vi "Receive mDNS Response.vi"(7 "timeout, ms (5000)":i32=5000, 8 "error in (no error)":errorcluster, 10 "query id":u16, 11 "connection ID":refnum<k16>) -> (0 "error out":errorcluster, 2 "response":T1 {"header"."response code" items=["NoError"=0, "FormErr"=1, "ServFail"=2, "NXDomain"=3, "NotImp"=4, "Refused"=5, "YXDomain"=6, "YXRRSet"=7, "NXRRSet"=8, "NotAuth"=9, "NotZone"=10, "DSOTYPENI"=11, "BADVERS/BADSIG"=16, "BADKEY"=17, "BADTIME"=18, "BADMODE"=19, "BADNAME"=20, "BADALG"=21, "BADTRUNC"=22, "BADCOOKIE"=23]; "header"."opcode" items=["Query"=0, "IQuery"=1, "Status"=2, "Notify"=4, "Update"=5, "DSO"=6]; "additional records"."class" items=["IN"=1, "CH"=3, "HS"=4]; "additional records"."type" items=["A"=1, "NS"=2, "MD"=3, "MF"=4, "CNAME"=5, "SOA"=6, "MB"=7, "MG"=8, "MR"=9, "NULL"=10, "WKS"=11, "PTR"=12, "HINFO"=13, "MINFO"=14, "MX"=15, "TXT"=16, "RP"=17, "AFSDB"=18, "X25"=19, "ISDN"=20, "RT"=21, "NSAP"=22, "NSAP-PTR"=23, "SIG"=24, "KEY"=25, "PX"=26, "GPOS"=27, "AAAA"=28, "LOC"=29, "NXT"=30, "EID"=31, "NIMLOC"=32, "SRV"=33, "ATMA"=34, "NAPTR"=35, "KX"=36, "CERT"=37, "A6"=38, "DNAME"=39, "SINK"=40, "OPT"=41, "APL"=42, "DS"=43, "SSHFP"=44, "IPSECKEY"=45, "RRSIG"=46, "NSEC"=47, "DNSKEY"=48, "DHCID"=49, "NSEC3"=50, "NSEC3PARAM"=51, "TLSA"=52, "SMIMEA"=53, "HIP"=55, "NINFO"=56, "RKEY"=57, "TALINK"=58, "CDS"=59, "CDNSKEY"=60, "OPENPGPKEY"=61, "CSYNC"=62, "ZONEMD"=63, "SVCB"=64, "HTTPS"=65, "SPF"=99, "UINFO"=100, "UID"=101, "GID"=102, "UNSPEC"=103, "NID"=104, "L32"=105, "L64"=106, "LP"=107, "EUI48"=108, "EUI64"=109, "URI"=256, "CAA"=257, "AVC"=258, "DOA"=259, "AMTRELAY"=260, "TA"=32768, "DLV"=32769]; "authority records"."class" items=["IN"=1, "CH"=3, "HS"=4]; "authority records"."type" items=["A"=1, "NS"=2, "MD"=3, "MF"=4, "CNAME"=5, "SOA"=6, "MB"=7, "MG"=8, "MR"=9, "NULL"=10, "WKS"=11, "PTR"=12, "HINFO"=13, "MINFO"=14, "MX"=15, "TXT"=16, "RP"=17, "AFSDB"=18, "X25"=19, "ISDN"=20, "RT"=21, "NSAP"=22, "NSAP-PTR"=23, "SIG"=24, "KEY"=25, "PX"=26, "GPOS"=27, "AAAA"=28, "LOC"=29, "NXT"=30, "EID"=31, "NIMLOC"=32, "SRV"=33, "ATMA"=34, "NAPTR"=35, "KX"=36, "CERT"=37, "A6"=38, "DNAME"=39, "SINK"=40, "OPT"=41, "APL"=42, "DS"=43, "SSHFP"=44, "IPSECKEY"=45, "RRSIG"=46, "NSEC"=47, "DNSKEY"=48, "DHCID"=49, "NSEC3"=50, "NSEC3PARAM"=51, "TLSA"=52, "SMIMEA"=53, "HIP"=55, "NINFO"=56, "RKEY"=57, "TALINK"=58, "CDS"=59, "CDNSKEY"=60, "OPENPGPKEY"=61, "CSYNC"=62, "ZONEMD"=63, "SVCB"=64, "HTTPS"=65, "SPF"=99, "UINFO"=100, "UID"=101, "GID"=102, "UNSPEC"=103, "NID"=104, "L32"=105, "L64"=106, "LP"=107, "EUI48"=108, "EUI64"=109, "URI"=256, "CAA"=257, "AVC"=258, "DOA"=259, "AMTRELAY"=260, "TA"=32768, "DLV"=32769]; "answers"."class" items=["IN"=1, "CH"=3, "HS"=4]; "answers"."type" items=["A"=1, "NS"=2, "MD"=3, "MF"=4, "CNAME"=5, "SOA"=6, "MB"=7, "MG"=8, "MR"=9, "NULL"=10, "WKS"=11, "PTR"=12, "HINFO"=13, "MINFO"=14, "MX"=15, "TXT"=16, "RP"=17, "AFSDB"=18, "X25"=19, "ISDN"=20, "RT"=21, "NSAP"=22, "NSAP-PTR"=23, "SIG"=24, "KEY"=25, "PX"=26, "GPOS"=27, "AAAA"=28, "LOC"=29, "NXT"=30, "EID"=31, "NIMLOC"=32, "SRV"=33, "ATMA"=34, "NAPTR"=35, "KX"=36, "CERT"=37, "A6"=38, "DNAME"=39, "SINK"=40, "OPT"=41, "APL"=42, "DS"=43, "SSHFP"=44, "IPSECKEY"=45, "RRSIG"=46, "NSEC"=47, "DNSKEY"=48, "DHCID"=49, "NSEC3"=50, "NSEC3PARAM"=51, "TLSA"=52, "SMIMEA"=53, "HIP"=55, "NINFO"=56, "RKEY"=57, "TALINK"=58, "CDS"=59, "CDNSKEY"=60, "OPENPGPKEY"=61, "CSYNC"=62, "ZONEMD"=63, "SVCB"=64, "HTTPS"=65, "SPF"=99, "UINFO"=100, "UID"=101, "GID"=102, "UNSPEC"=103, "NID"=104, "L32"=105, "L64"=106, "LP"=107, "EUI48"=108, "EUI64"=109, "URI"=256, "CAA"=257, "AVC"=258, "DOA"=259, "AMTRELAY"=260, "TA"=32768, "DLV"=32769]}, 3 "connection ID out":refnum<k16>)   [LabVIEW 2015, in "PL DNS Client.lvlib"]
doc: "Receives Multicast DNS response for specified <b>query id</b> using specified <b>connection ID</b>."
uses:
  PL DNS Client.lvlib
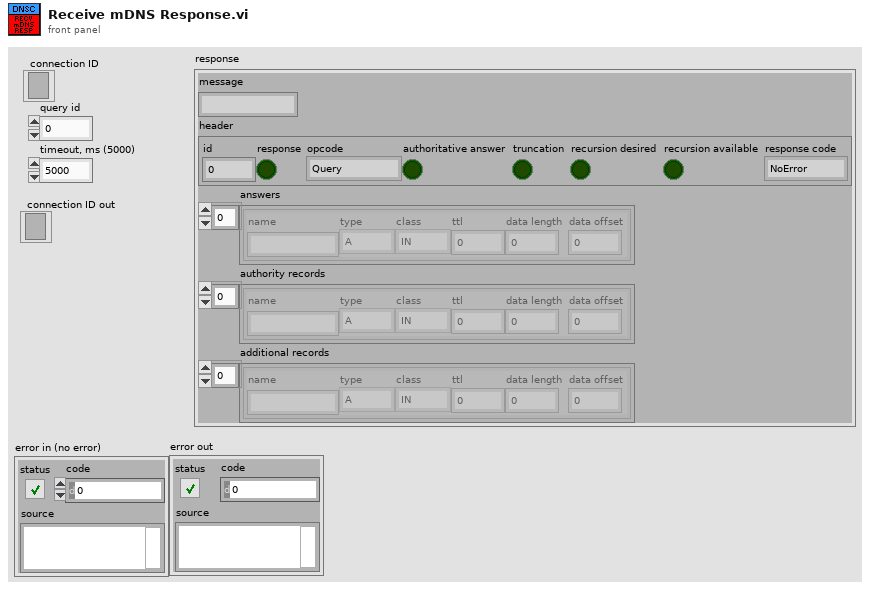
[diagram p1: front panel]
types:
  T1 = cluster{"message":string, "header":cluster{"id":u16, "response":bool, "opcode":u8, "authoritative answer":bool, "truncation":bool, "recursion desired":bool, "recursion available":bool, "response code":u16}, "answers":cluster{"name":string, "type":u16, "class":u16, "ttl":u32, "data length":u16, "data offset":u16}[], "authority records":cluster{"name":string, "type":u16, "class":u16, "ttl":u32, "data length":u16, "data offset":u16}[], "additional records":cluster{"name":string, "type":u16, "class":u16, "ttl":u32, "data length":u16, "data offset":u16}[]}
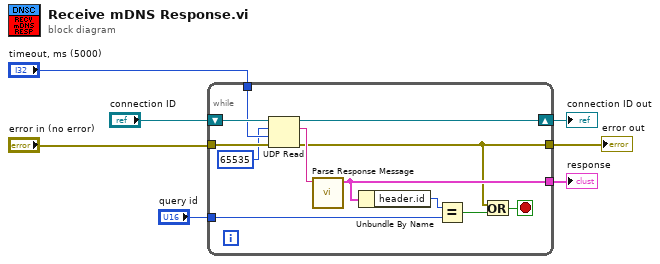
[diagram p0: block diagram]
diagram:
  n1 = while {
    tunnel: "error in (no error)" -> [w13]
    tunnel: "timeout, ms (5000)" -> [w18]
    shift-right: [w14] -> w2
    shift-left: "connection ID" -> [w19]
    tunnel: [w17] -> w6
    tunnel: [w8] -> w1
    tunnel: "query id" -> [w12]
    stop <- w16 stop-if-true
    n2 = UDP Read(connection ID=w19, max size (548)=65535, timeout ms (25000)=w18, 8:w13) -> (data out=w15:string, error out=w8:errorcluster, 3:w14:refnum<k16>)  [unwired: 2 out]
    n3 = call "Parse Response Message.vi"("message"=w15) -> ("response"=w17:T1)  [unwired: 10 in]
    n4 = Unbundle By Name(w17) -> ("header.id"=w9:u16)
    n5 = Equal?(x=w9, y=w12) -> (x = y?=w10:bool)
    n6 = Or(x=w8, y=w10) -> (x .or. y?=w16:bool)
  }
  "response" <- w6
  "connection ID out" <- w2
  "error out" <- w1
